vi "Generate Simulated Data.vi"(7 "Type de mode":bool, 8 "error in (no error)":T2 caption="entrée d'erreur (pas d'erreur)", 9 "Péri":tag="Dev1", 10 "Longueur d'onde":dbl, 11 "Type de signal":T1) -> (0 "error out":T2 caption="sortie d'erreur", 2 "Données du graphe":waveform(dbl)[](array[waveform]))   [LabVIEW 2018, in "Acquisition.lvlib"]
doc: "Génère des exemples de waveforms en fonction du type de signal dans l'entrée Configuration du matériel."
uses:
  Acquisition.lvlib
  Signal Type.ctl
  <vilib>/Analysis/baseanly.llb/Mean (DBL).vi
  <vilib>/Analysis/NI_AALBase.lvlib
panel:
  out "Graphe déroulant":dynamicdata(graph)
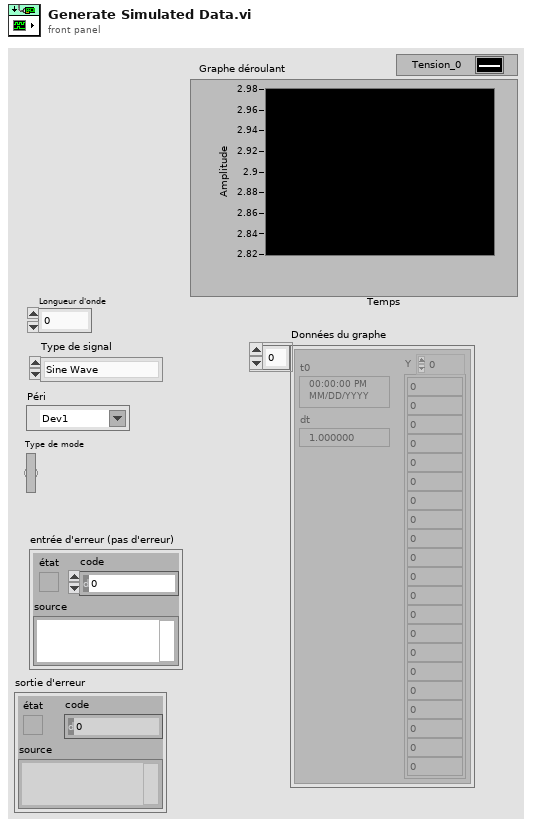
[diagram p1: front panel]
types:
  T1 = typedef "Acquisition.lvlib/Signal Type.ctl" = enum16{"Sine Wave", "Square with Noise", "Signal triangulaire", "Simulation DAQ"}
  T2 = cluster{"état":bool, "code":i32, "source":string}
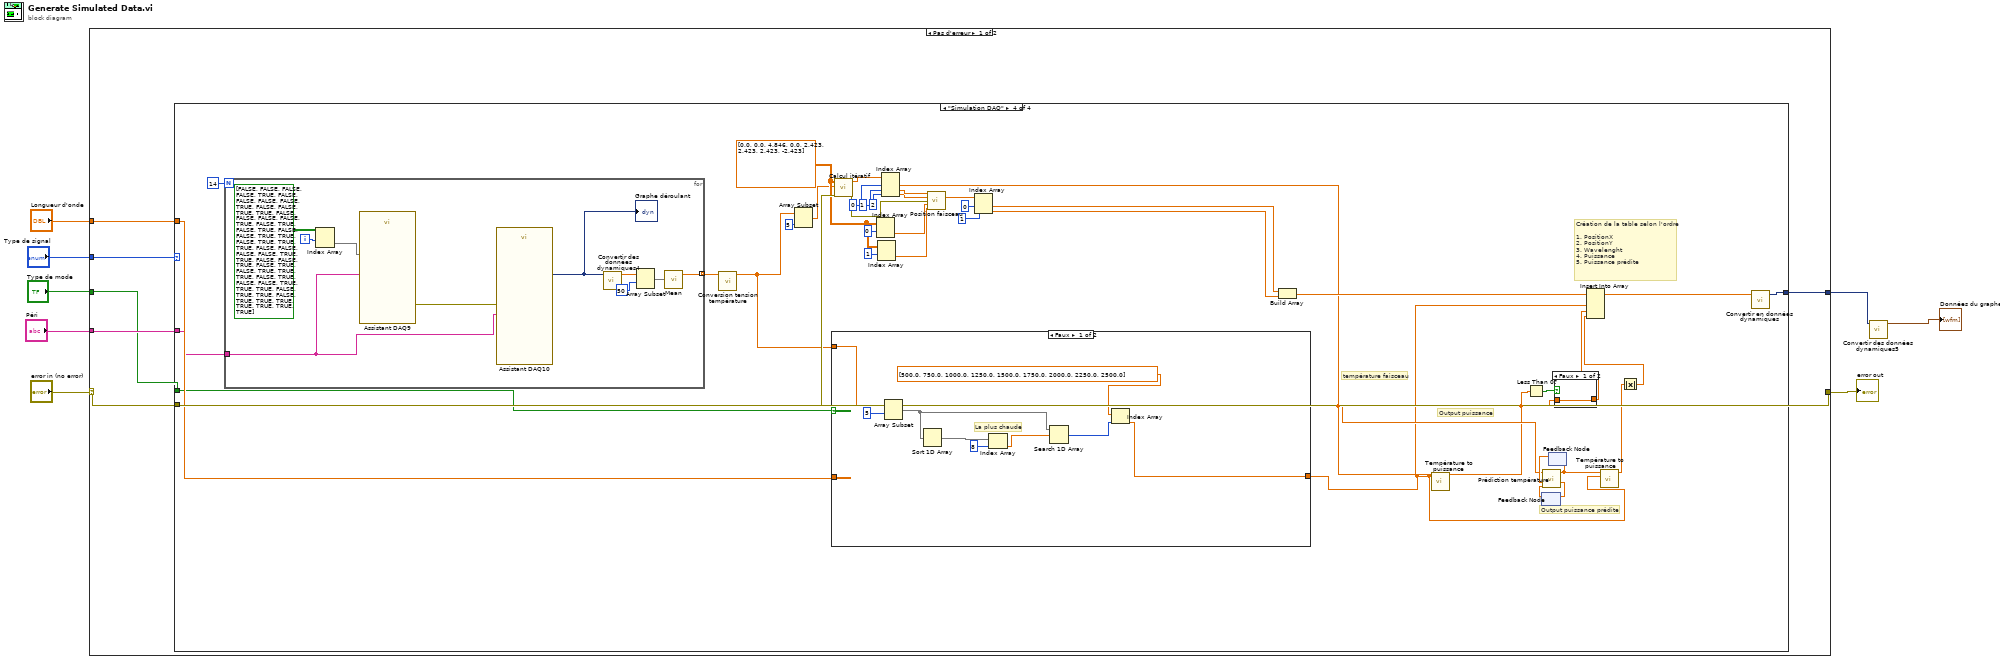
[diagram p0: block diagram]
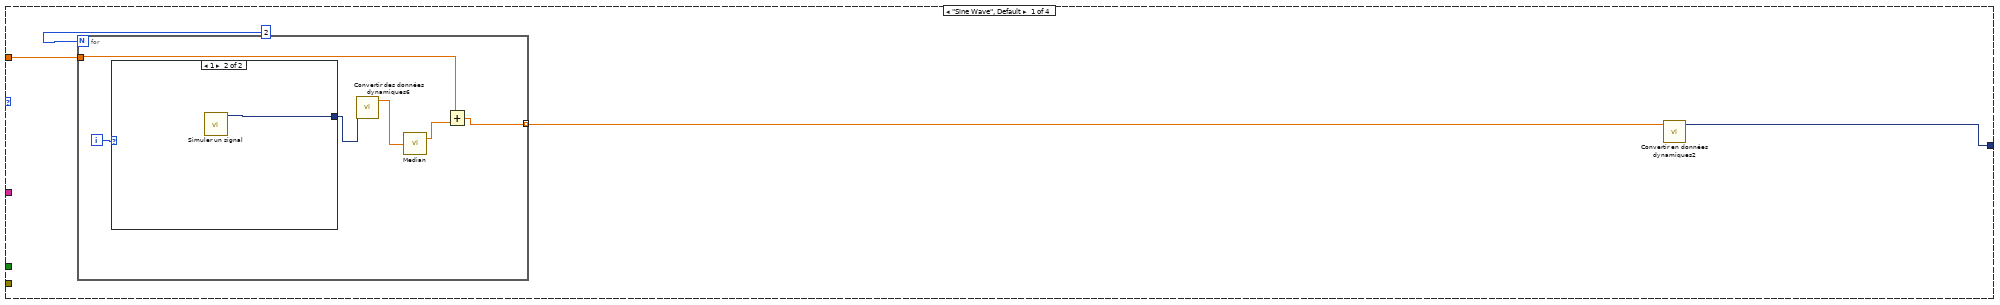
[diagram p2: hidden frame]
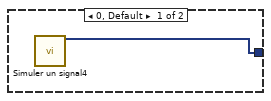
[diagram p3: hidden frame]
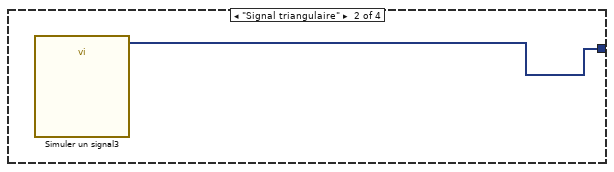
[diagram p4: hidden frame]
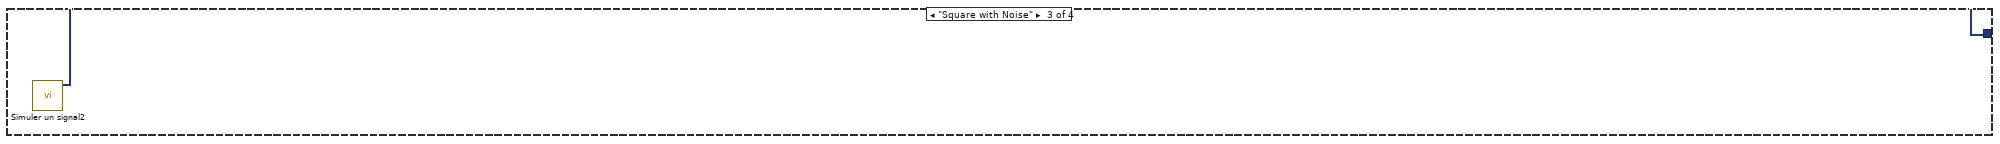
[diagram p5: hidden frame]
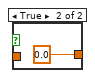
[diagram p6: hidden frame]
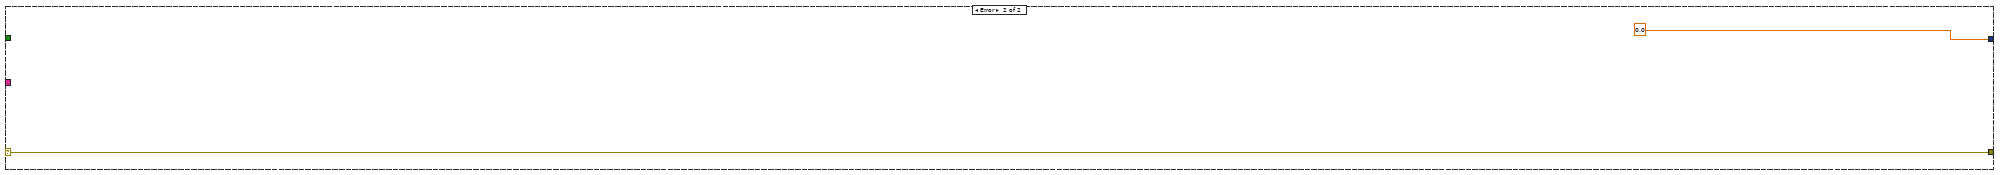
[diagram p8: hidden frame]
diagram:
  n1 = case shown="Pas d'erreur" "error in (no error)" {
    selector: "error in (no error)" -> [w9 w92]
    tunnel: [w9 w92] -> w7
    tunnel: "Type de signal" -> [w14 _]
    tunnel: [w13 0.0] -> w4
    tunnel: "Longueur d'onde" -> [w12 _]
    tunnel: "Péri" -> [w11 _]
    tunnel: "Type de mode" -> [w10 _]
    frame No Error {
      n2 = case shown="\"Simulation DAQ\"" w14 {
        tunnel: [w17 w27 w28 w67] -> w13
        tunnel: w12 -> [w16 _ _ w66]
        tunnel: w11 -> [_ _ _ w65]
        tunnel: w10 -> [_ _ _ w64]
        tunnel: w9 -> [_ _ _ w61]
        frame "Sine Wave", Default {
          n3 = for {
            N: 2 -> [_]
            tunnel: [w20] -> w15 mode=indexing
            tunnel: w16 -> [w19]
            i -> [w24]
            n4 = case shown="1" w24 {
              tunnel: [w25 w26] -> w23
              frame 0, Default {
                n5 = call "Simuler un signal4"() -> ("CC"=w25:dynamicdata)  [unwired: 14 in, 1 out]
              }
              frame 1 {
                n6 = call "Simuler un signal"() -> ("Sinus avec Bruit uniforme"=w26:dynamicdata)  [unwired: 14 in, 1 out]
              }
            }
            n7 = call "Convertir des données dynamiques6"("Dynamic Data Type"=w23) -> ("Array"=w22:dbl[])  [unwired: 3 in]
            n8 = call <vilib>:"Median.vi"("X"=w22) -> ("median"=w21:dbl)  [unwired: 1 out]
            n9 = Add(x=w19, y=w21) -> (x+y=w20:dbl)
          }
          n10 = call "Convertir en données dynamiques2"("Array"=w15) -> ("Dynamic Data Type"=w17:dynamicdata)  [unwired: 3 in]
        }
        frame "Signal triangulaire" {
          n11 = call "Simuler un signal3"() -> ("Triangle"=w27:dynamicdata)  [unwired: 14 in, 1 out]
        }
        frame "Square with Noise" {
          n12 = call "Simuler un signal2"() -> ("Square with Gaussian Noise"=w28:dynamicdata)  [unwired: 14 in, 1 out]
        }
        frame "Simulation DAQ" {
          w60 = dbl[][] [[0.0, 0.0], [4.846, 0.0], [2.423, 2.423], [2.423, -2.423]] ("Position des capteurs")
          # "température faisceau"
          # "Output puissance prédite"
          # "Création de la table selon l'ordre\n\n1. PositionX\n2. PositionY\n3. Wavelenght\n4. Puissance\n5. Puissance prédite"
          # "Output puissance"
          n13 = for {
            N: 14 -> [_]
            tunnel: [w82] -> w62 mode=indexing
            tunnel: w65 -> [w81]
            i -> [w88]
            n14 = Index Array(array=bool[][] [[FALSE, FALSE, FALSE, FALSE], [TRUE, FALSE, FALSE, FALSE], [FALSE, TRUE, FALSE, FALSE], [TRUE, TRUE, FALSE, FALSE], [FALSE, FALSE, TRUE, FALSE], [TRUE, FALSE, TRUE, FALSE], [FALSE, TRUE, TRUE, FALSE], [TRUE, TRUE, TRUE, FALSE], [FALSE, FALSE, FALSE, TRUE], [TRUE, FALSE, FALSE, TRUE], [FALSE, TRUE, FALSE, TRUE], [TRUE, TRUE, FALSE, TRUE], [FALSE, FALSE, TRUE, TRUE], [TRUE, FALSE, TRUE, TRUE], [FALSE, TRUE, TRUE, TRUE], [TRUE, TRUE, TRUE, TRUE]], index (row)=w88) -> (element=w87:bool[])  [unwired: 1 in]
            n15 = call "Assistant DAQ9"("data"=w87, "nom du périphérique"=w81) -> ("error out"=w90:errorcluster)  [unwired: 16 in, 1 out]
            n16 = call "Assistant DAQ10"("error in"=w90, "nom du périphérique"=w81) -> ("data"=w86:dynamicdata)  [unwired: 15 in, 2 out]
            "Graphe déroulant" <- w86
            n17 = call "Convertir des données dynamiques4"("Dynamic Data Type"=w86) -> ("Array"=w85:dbl[])  [unwired: 3 in]
            n18 = Array Subset(array=w85, index=50 ("indice")) -> (w83:dbl[])  [unwired: 1 in]
            n19 = call-poly <vilib>:"Mean.vi"("X"=w83) -> ("mean"=w82:dbl)  [unwired: 1 out]
          }
          n20 = call "Conversion tension température.vi"("Tension In"=w62) -> ("Température Out"=w32:dbl[])  [unwired: 10 in]
          n21 = Array Subset(array=w32, length=5 ("longueur")) -> (w36:dbl[])  [unwired: 1 in]
          n22 = case shown="Faux" w64 {
            tunnel: [w71 w80] -> w35
            tunnel: w66 -> [_ w80]
            tunnel: w32 -> [w79 _]
            frame False {
              # "La plus chaude"
              n23 = Array Subset(array=w79, index=5 ("indice")) -> (w74:dbl[])  [unwired: 1 in]
              n24 = Sort 1D Array(array=w74) -> (sorted array=w76:dbl[])
              n25 = Index Array(array=w76, index=8 ("indice")) -> (element=w75:dbl)
              n26 = Search 1D Array(1D array=w74, element=w75) -> (index of element=w73:i32)  [unwired: 1 in]
              n27 = Index Array(array=dbl[] [500.0, 750.0, 1000.0, 1250.0, 1500.0, 1750.0, 2000.0, 2250.0, 2500.0], index=w73) -> (element=w71:dbl)
            }
            frame True {
            }
          }
          n28 = call "Calcul itératif.vi"("error in (no error)"=w61, "Température capteur 1-2-3-4-Ambiant"=w36, "Position des capteurs"=w60) -> ("error out"=w43:T2, "DATA - T/R1/R2/R3"=w47:dbl[])  [unwired: 7 in]
          n29 = Index Array(array=w60, index (row)=0 ("indice (ligne)")) -> (element=w59:dbl[])  [unwired: 1 in]
          n30 = Index Array(array=w60, index (row)=1 ("indice (ligne)")) -> (element=w58:dbl[])  [unwired: 1 in]
          n31 = Index Array(array=w47, index #1=0, index #2=1 ("indice"), index #3=2 ("indice")) -> (element #1=w39:dbl, element #2=w46:dbl, element #3=w45:dbl)
          n32 = call "Position faisceau.vi"("R1"=w46, "R2"=w45, "error in (no error)"=w43, "Capteur 1"=w59, "Capteur 2"=w58) -> ("Coord"=w55:dbl[])  [unwired: 9 in, 1 out]
          n33 = Index Array(array=w55, index #1=0 ("indice"), index #2=1 ("indice")) -> (element #1=w52:dbl, element #2=w51:dbl)
          n34 = Build Array(w52, w51) -> (w44:dbl[])
          n35 = call "Température to puissance.vi"("Longueur d'onde"=w35, "Température max"=w39) -> ("Puissance"=w30:dbl)  [unwired: 9 in]
          n36 = Less Than 0?(x=w30) -> (x < 0?=w31:bool)
          n37 = feedback #1() -> (w42:dbl)  [unwired: 1 in]
          n38 = feedback #2() -> (w41:dbl)  [unwired: 1 in]
          n39 = call "Prédiction température.vi"("Temps -2"=w42, "Temps -1"=w41, "Temps 0"=w39) -> ("Temps-1"=w40:dbl, "Temps pred"=w38:dbl)  [unwired: 7 in]
          n40 = feedback-in #1(w40) -> ()
          n41 = feedback-in #2(w38) -> ()
          n42 = case shown="Faux" w31 {
            tunnel: [w69 0.0] -> w29
            tunnel: w30 -> [w69 _]
            frame False {
            }
            frame True {
            }
          }
          n43 = call "Température to puissance.vi"("Longueur d'onde"=w35, "Température max"=w38) -> ("Puissance"=w34:dbl)  [unwired: 9 in]
          n44 = Absolute Value(x=w34) -> (abs(x)=w33:dbl)
          n45 = Insert Into Array(array=w44, new element #1=w35, new element #2=w29, new element #3=w33) -> (w63:dbl[])  [unwired: 1 in]
          n46 = call "Convertir en données dynamiques"("Array"=w63) -> ("Dynamic Data Type"=w67:dynamicdata)  [unwired: 3 in]
        }
      }
    }
    frame Error {
    }
  }
  "error out" <- w7
  n47 = call "Convertir des données dynamiques5"("Dynamic Data Type"=w4) -> ("Array of Waveform"=→"Données du graphe":waveform(dbl)[])  [unwired: 3 in]
